vi "Read Output.vi"   [LabVIEW 2010, in "Agilent U2722.lvlib"]
doc: "Returns the measurements from a desired channel."
uses:
  Agilent U2722.lvlib
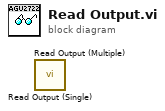
[diagram p0: block diagram]
diagram:
  n1 = call "Read Output (Single).vi"() -> ()  [unwired: 8 in, 4 out]
  n2 = call "Read Output (Multiple).vi"() -> ()  [unwired: 8 in, 4 out]
